vi "Reshape Array to 1D VArray.vi"(8 "error in (no error)":errorcluster, 10 "MultiD Array":variant) -> (0 "error out":errorcluster, 1 "Size(s)":u32[](array[numeric]), 2 "1D VArray":variant)   [LabVIEW 2012, in "TD Tools.lvlib"]
uses:
  TD Tools.lvlib
  <userlib>/_OpenG.lib/lvdata/lvdata.llb/Type Descriptor Enumeration__ogtk.ctl
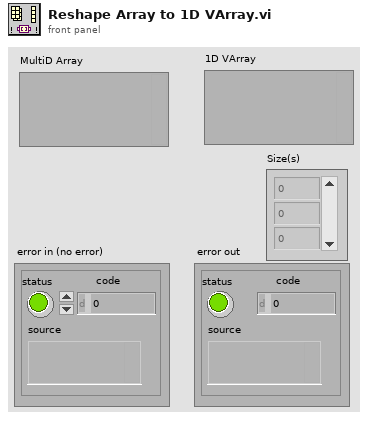
[diagram p1: front panel]
types:
  T1 = typedef "Type Descriptor Enumeration__ogtk.ctl" = enum8{"<Null>", "I8", "I16", "I32", "I64", "U8", "U16", "U32", "U64", "SGL", "DBL", "EXT", "CSG", "CDB", "CXT", "0x0F", "0x10", "0x11", "0x12", "0x13", "0x14", "Enum U8", "Enum U16", "Enum U32", "Enum U64", "SGL PQ", "DBL PQ", "EXT PQ", "CSG PQ", "CDB PQ", "CXT PQ", "0x1F", "0x20", "Boolean", "0x22", "0x23", "0x24", "0x25", "0x26", "0x27", "0x28", "0x29", "0x2A", "0x2B", "0x2C", "0x2D", "0x2E", "0x2F", "String", "0x31", "Path", "Pict", "0x34", "0x35", "0x36", "DAQ", "0x38", "0x39", "0x3A", "0x3B", "0x3C", "0x3D", "0x3E", "0x3F", "Array", "0x41", "0x42", "0x43", "0x44", "0x45", "0x46", "0x47", "0x48", "0x49", "0x4A", "0x4B", "0x4C", "0x4D", "0x4E", "0x4F", "Cluster", "0x51", "0x52", "Variant", "Waveform", "0x55", "0x56", "0x57", "0x58", "0x59", "0x5A", "0x5B", "0x5C", "0x5D", "0x5E", "0x5F", "0x60", "0x61", "0x62", "0x63", "0x64", "0x65", "0x66", "0x67", "0x68", "0x69", "0x6A", "0x6B", "0x6C", "0x6D", "0x6E", "0x6F", "Refnum"}
  T2 = typedef "TD Tools.lvlib/Type Descriptor.ctl" = u16[]
  T3 = typedef "TD Tools.lvlib/Type Descriptor Header.ctl" = cluster{"length":u16, "private":u8, "type":T4, "# elements":u16}
  T4 = typedef "TD Tools.lvlib/Type Descriptor Enumeration.ctl" = enum16{"<Null>", "I8", "I16", "I32", "I64", "U8", "U16", "U32", "U64", "SGL", "DBL", "EXT", "CSG", "CDB", "CXT", "0x0F", "0x10", "0x11", "0x12", "0x13", "0x14", "Enum U8", "Enum U16", "Enum U32", "Enum U64", "SGL PQ", "DBL PQ", "EXT PQ", "CSG PQ", "CDB PQ", "CXT PQ", "0x1F", "0x20", "Boolean", "0x22", "0x23", "0x24", "0x25", "0x26", "0x27", "0x28", "0x29", "0x2A", "0x2B", "0x2C", "0x2D", "0x2E", "0x2F", "String", "0x31", "Path", "Pict", "0x34", "0x35", "0x36", "DAQ", "0x38", "0x39", "0x3A", "0x3B", "0x3C", "0x3D", "0x3E", "0x3F", "Array", "0x41", "0x42", "0x43", "0x44", "0x45", "0x46", "0x47", "0x48", "0x49", "0x4A", "0x4B", "0x4C", "0x4D", "0x4E", "0x4F", "Cluster", "0x51", "0x52", "Variant", "Waveform", "0x55", "0x56", "0x57", "0x58", "0x59", "0x5A", "0x5B", "0x5C", "0x5D", "0x5E", "0x5F", "0x60", "0x61", "0x62", "0x63", "0x64", "0x65", "0x66", "0x67", "0x68", "0x69", "0x6A", "0x6B", "0x6C", "0x6D", "0x6E", "0x6F", "Refnum"}
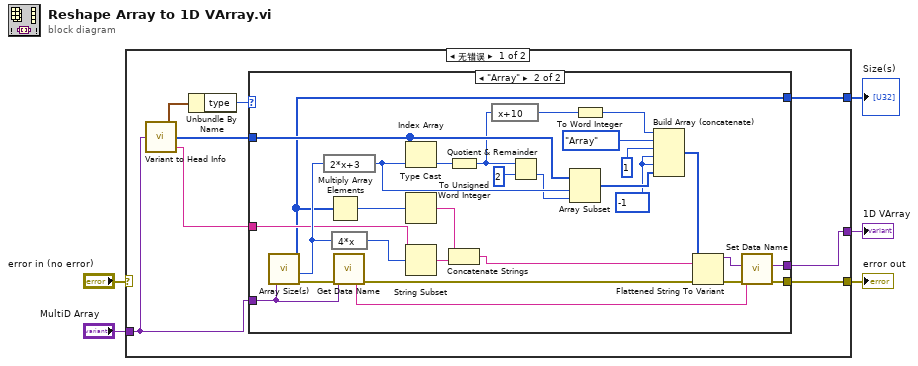
[diagram p0: block diagram]
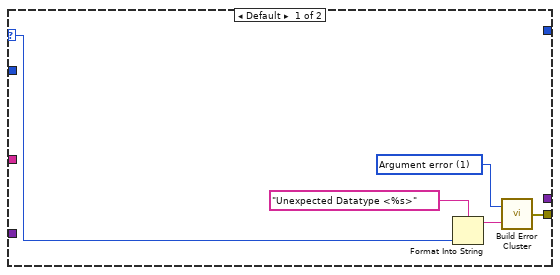
[diagram p2: hidden frame]
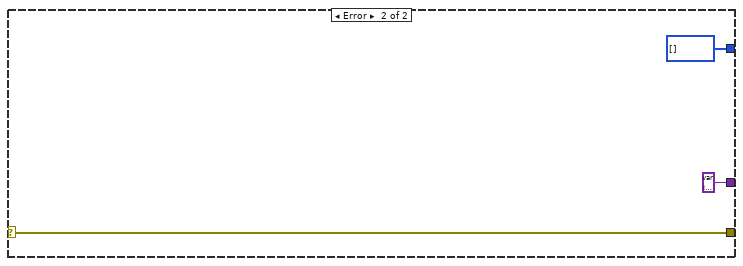
[diagram p3: hidden frame]
diagram:
  n1 = case shown="无错误" "error in (no error)" {
    selector: "error in (no error)" -> [_ w50]
    tunnel: [w13 w50] -> w2
    tunnel: [w8 variant ("Variant")] -> w4
    tunnel: [w7 u32[] [] ("Size(s)")] -> w1
    tunnel: "MultiD Array" -> [w6 _]
    frame No Error {
      n2 = call "Variant to Head Info.vi"("Variant"=w6) -> ("Data String"=w9:string, "Type Descriptor"=w10:T2, "Type Descriptor Header"=w12:T3)  [unwired: 2 in]
      n3 = Unbundle By Name(w12) -> ("type"=w11:T4)
      n4 = case shown="\"Array\"" w11 {
        selector: w11 -> [w16 _]
        tunnel: [w18 w26] -> w13
        tunnel: w10 -> [_ w45]
        tunnel: w9 -> [_ w37]
        tunnel: w6 -> [_ w24]
        tunnel: [_ w28] -> w8
        tunnel: [_ w30] -> w7
        frame Default {
          w17 = 1 items=["No error", "Argument error", "Memory is full", "Out of zone", "End of file", "File already open", "Generic file I/O error", "File not found", "File permission error", "Disk is full", "Duplicate path", "Too many files open", "System feature not enabled", "Resource file not found", "Cannot add resource", "Resource not found", "Image not found", "Image memory error", "Pen does not exist", "Config type invalid", "Config token not found", "Config parse error", "Config memory error", "Bad external code format", "Bad external code offset", "External code not present", "Null window", "Destroy window error", "Null menu", "Print aborted", "Bad print record", "Print driver error", "Windows error during printing", "Memory error during printing", "Print dialog error", "Generic print error", "Invalid device refnum", "Device not found", "Device parameter error", "Device unit error", "Cannot open device", "Device call aborted", "Generic error", "Cancelled by user", "Object ID too low", "Object ID too high", "Object not in heap", "Unknown heap", "Unknown object (invalid DefProc)", "Unknown object (DefProc not in table)", "Message out of range", "Invalid (null) method", "Unknown message", "Manager call not supported", "Bad address", "Network operation in progress", "Network operation timed out", "Connection is busy", "Network attribute not supported", "Network error", "Address in use", "System out of memory", "Connection aborted", "Connection refused", "Not connected", "Already connected", "Connection closed", "Initialization error (interapplication manager)", "Bad occurrence", "Wait on unbound occurrence handler", "Occurrence queue overflow", "Datalog type conflict", "Unused", "Unrecognized type (interapplication manager)", "Memory corrupt", "Failed to make temporary DLL", "Old CIN version", "Drag socket not found", "Failed to load drop-object", "Failed to register OLE object", "Failed to release OLE object", "Format specifier type mismatch", "Unknown format specifier", "Too few format specifiers", "Too many format specifiers", "Scan failed", "Newer CIN version", "Error converting to variant", "Runtime menu error", "Password tampered", "Variant attribute not found", "Incompatible variant data type", "Event data is not available", "Event Store is not present", "Occurrence is not found", "Event Queue is not created", "Event info is not available", "Refnum passed is NULL", "Error retrieving Class GUID", "Error retrieving CoClass GUID", "Error retrieving TypeLib GUID.", "Bad built application magic bytes.", "Specific driver is different from the specific driver associated with the Logical Name.", "There is no session opened to the class driver.", "Max Error", "MAX - Error with config objects", "MAX - Error loading configuration", "MAX - Group not supported"]
          n5 = Format Into String(format string="Unexpected Datatype <%s>" ("Format String"), w16) -> (resulting string=w14:string)  [unwired: 2 in, 1 out]
          n6 = call "Build Error Cluster.vi"("String to Prepend to source (\"\")"=w14, "code"=w17) -> ("error out"=w18:errorcluster)
        }
        frame "Array" {
          w39 = i16 -1 ("Input Element")
          n7 = call "Array Size(s).vi"("Array"=w24) -> ("错误输出"=w23:errorcluster, "N dims"=w38:u32, "Size(s)"=w30:u32[])  [unwired: 8 in]
          n8 = expression code="2*x+3"(w38) -> (w47:u32)
          n9 = Multiply Array Elements(1:w30) -> (0:w35:u32)
          n10 = expression code="4*x"(w38) -> (w36:u32)
          n11 = call "Get Data Name.vi"("错误输入"=w23, "Data"=w24) -> ("错误输出"=w22:errorcluster, "Data Name"=w25:string)  [unwired: 7 in, 1 out]
          n12 = Index Array(array=w45, index=w47) -> (element=w40:u16)
          n13 = Type Cast(x=w35) -> (*(type *) &x=w34:string)  [unwired: 1 in]
          n14 = String Subset(string=w37, offset (0)=w36) -> (substring=w33:string)  [unwired: 1 in]
          n15 = To Unsigned Word Integer(number=w40) -> (unsigned 16bit integer=w21:u16)
          n16 = Concatenate Strings(w34, w33) -> (w31:string)
          n17 = expression code="x+10"(w21) -> (w42:u16)
          n18 = Quotient & Remainder(x=w21, y=u16 2) -> (floor(x/y)=w41:u16)  [unwired: 1 out]
          n19 = Array Subset(array=w45, index=w47, length=w41) -> (w44:T2)
          n20 = To Word Integer(number=w42) -> (16bit integer=w20:i16)
          n21 = Build Array (concatenate)(w20, Type_Descriptor_Enumeration__ogtk."Array" ("Type Descriptor Enumeration"), i16 1 ("Dim 1D"), w39, w39, w44) -> (w32:T2)
          n22 = Flattened String To Variant(4:w22, 6:w31, 7:w32) -> (0:w27:errorcluster, 3:w29:variant)
          n23 = call "Set Data Name.vi"("错误输入"=w27, "Data Name"=w25, "Data"=w29) -> ("错误输出"=w26:errorcluster, "Renamed Data"=w28:variant)  [unwired: 7 in]
        }
      }
    }
    frame Error {
    }
  }
  "error out" <- w2
  "1D VArray" <- w4
  "Size(s)" <- w1
